vi "TempSoak_Read.vi"(0 "VISA":refnum<visa-resource-name>="TCPIP0::169.254.70.190::502::SOCKET", 1 "connection ID":refnum<k5>, 5 "error in (no error)":errorcluster, 7 "Wait(min)":dbl, 9 "stop":bool, 13 "CloseTcp(t)":bool=TRUE) -> (12 "Waveform Chart":cluster{"Value":sgl, "Value":sgl}(graph)={"Value"=27.280333, "Value"=26.223886} caption="Done!!!", 14 "visa out":refnum<visa-resource-name>, 15 "connection ID out":refnum<k5>, 19 "error out":errorcluster)   [LabVIEW 2018]
panel:
  out "x/y":dbl
  out "x-y":dbl=15.43812059999982
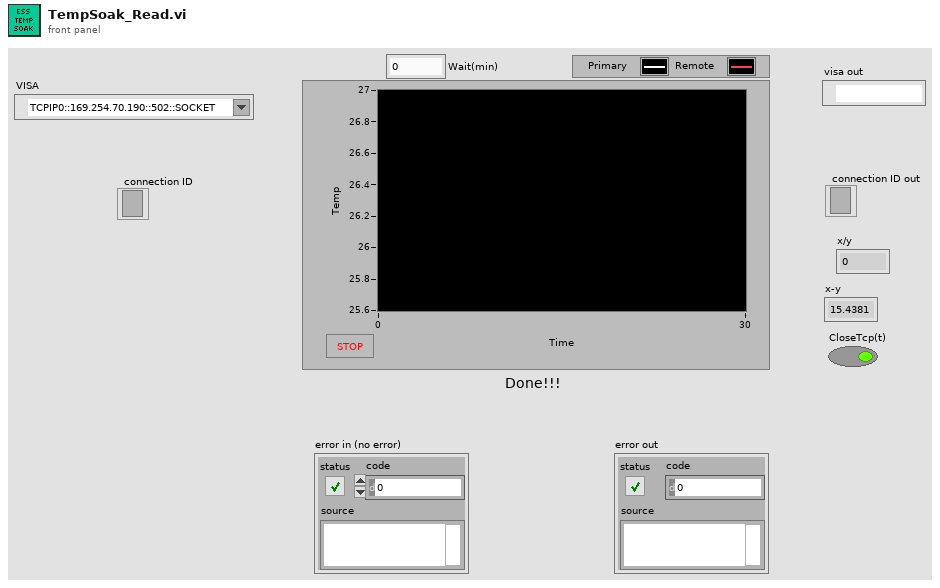
[diagram p1: front panel]
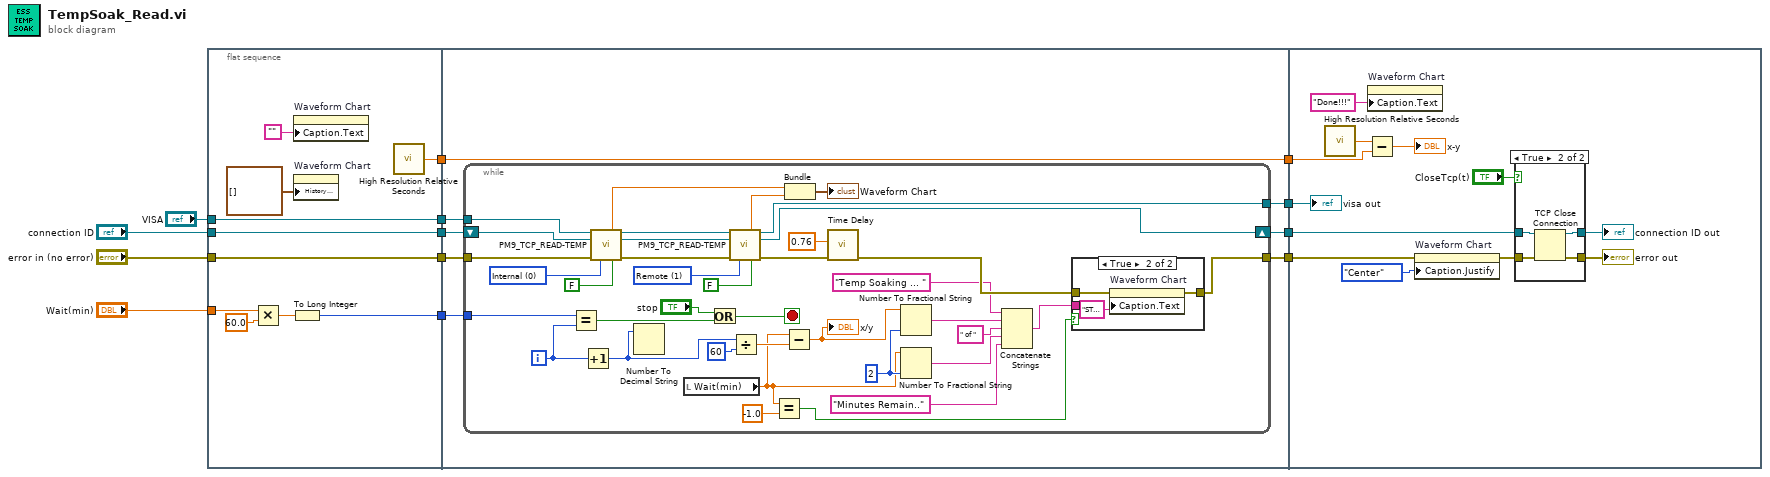
[diagram p0: block diagram]
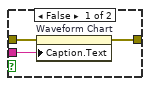
[diagram p2: hidden frame]
diagram:
  n1 = flat-sequence {
    tunnel: "connection ID" -> [w22]
    tunnel: "VISA" -> [w23]
    tunnel: [w23] -> w11
    tunnel: [w22] -> w10
    tunnel: [w21] -> w9
    tunnel: [w20] -> w7
    tunnel: "error in (no error)" -> [w20]
    tunnel: "Wait(min)" -> [w19]
    tunnel: [w16] -> w2
    tunnel: w11 -> [w31]
    tunnel: w10 -> [w30]
    tunnel: w9 -> [w29]
    tunnel: [w29] -> w8
    tunnel: w7 -> [w28]
    tunnel: [w27] -> w6
    tunnel: [w26] -> w4
    tunnel: w2 -> [w25]
    tunnel: [w24] -> w1
    tunnel: w8 -> [w86]
    tunnel: w6 -> [w80]
    tunnel: w4 -> [w84]
    tunnel: w1 -> [w76]
    frame #0 {
      n2 = Multiply(x=w19, y=60.0) -> (x*y=w17:dbl)
      n3 = To Long Integer(number=w17) -> (32bit integer=w16:i32)
      n4 = property on="Waveform Chart" class="WFChart (strict)"("Caption.Text"="") -> ()  [unwired: 2 in, 2 out]
      n5 = property on="Waveform Chart" class="WFChart (strict)"("History Data"=cluster{"Value":sgl, "Value":sgl}[] []) -> ()  [unwired: 2 in, 2 out]
      n6 = call <vilib>:"High Resolution Relative Seconds.vi"() -> ("relative seconds"=w21:dbl)
    }
    frame #1 {
      n7 = while {
        tunnel: w31 -> [w69]
        tunnel: [w62] -> w24
        shift-right: [w58] -> w26
        shift-left: w30 -> [w57]
        tunnel: w28 -> [w55]
        tunnel: [w48] -> w27
        tunnel: w25 -> [w52]
        i -> [w46]
        stop <- w51 stop-if-true
        w35 = i16 2 ("precision (6)")
        w64 = u16 1 items=["Internal", "Remote"] ("Sensor")
        w65 = u16 0 items=["Internal", "Remote"] ("Sensor")
        n8 = Equal?(x=w52, y=w46) -> (x = y?=w50:bool)
        n9 = Increment(x=w46) -> (x+1=w44:i32)
        n10 = call "PM9_TCP_READ-TEMP.vi"("VISA"=w69, "connection ID"=w57, "error in (no error)"=w55, "Sensor"=w65, "Close tcp(t)"=FALSE) -> ("Value"=w61:sgl, "visa out"=w63:refnum<visa-resource-name>, "connection ID out"=w68:refnum<k5>, "error out"=w54:errorcluster)  [unwired: 7 in]
        n11 = Number To Decimal String(number=w44) -> ()  [unwired: 1 in, 1 out]
        n12 = local read "Wait(min)"() -> (w33:dbl)
        n13 = Or(x="stop", y=w50) -> (x .or. y?=w51:bool)
        n14 = call "PM9_TCP_READ-TEMP.vi"("VISA"=w63, "connection ID"=w68, "error in (no error)"=w54, "Sensor"=w64, "Close tcp(t)"=FALSE) -> ("Value"=w60:sgl, "visa out"=w62:refnum<visa-resource-name>, "connection ID out"=w58:refnum<k5>, "error out"=w53:errorcluster)  [unwired: 7 in]
        n15 = Divide(x=w44, y=60) -> (x/y=w42:dbl)
        n16 = Equal?(x=w33, y=-1.0) -> (x = y?=w34:bool)
        n17 = Subtract(x=w33, y=w42) -> (x-y=w41:dbl)
        "x/y" <- w41
        n18 = Bundle("Value"=w61, "Value"=w60) -> (→"Waveform Chart":cluster{"Value":sgl, "Value":sgl})  [unwired: 1 in]
        n19 = call "Time Delay"("error in (no error)"=w53, "Delay Time (s)"=0.76 ("milliseconds to wait")) -> ("error out"=w49:errorcluster)  [unwired: 9 in]
        n20 = Number To Fractional String(number=w41, precision (6)=w35) -> (F-format string=w40:string)  [unwired: 2 in]
        n21 = Number To Fractional String(number=w33, precision (6)=w35) -> (F-format string=w38:string)  [unwired: 2 in]
        n22 = Concatenate Strings("Temp Soaking ... ", w40, " of " ("string"), w38, "Minutes Remain.." ("string")) -> (w36:string)
        n23 = case shown="True" w34 {
          tunnel: w49 -> [w72 w75]
          tunnel: [w71 w74] -> w48
          tunnel: w36 -> [w70 _]
          frame False {
            n24 = property on="Waveform Chart" class="WFChart (strict)"(error in=w72, "Caption.Text"=w70) -> (error out=w71:errorcluster)  [unwired: 1 in, 1 out]
          }
          frame True {
            n25 = property on="Waveform Chart" class="WFChart (strict)"(error in=w75, "Caption.Text"="STOP to Cancel" ("string")) -> (error out=w74:errorcluster)  [unwired: 1 in, 1 out]
          }
        }
      }
    }
    frame #2 {
      n26 = call <vilib>:"High Resolution Relative Seconds.vi"() -> ("relative seconds"=w87:dbl)
      n27 = Subtract(x=w87, y=w86) -> (x-y=→"x-y":dbl)
      n28 = property on="Waveform Chart" class="WFChart (strict)"("Caption.Text"="Done!!!") -> ()  [unwired: 2 in, 2 out]
      n29 = property on="Waveform Chart" class="WFChart (strict)"(error in=w80, "Caption.Justify"=enum16{"Left", "Center", "Right"}."Center" ("Caption.Justification")) -> (error out=w79:errorcluster)  [unwired: 1 in, 1 out]
      n30 = case shown="True" "CloseTcp(t)" {
        tunnel: w84 -> [w89 w93]
        tunnel: [w89 w92] -> w83
        tunnel: [w88 w91] -> w82
        tunnel: w79 -> [w88 w90]
        frame False {
        }
        frame True {
          n31 = TCP Close Connection(connection ID=w93, error in (no error)=w90) -> (connection ID out=w92:refnum<k5>, error out=w91:errorcluster)  [unwired: 1 in]
        }
      }
      "error out" <- w82
      "connection ID out" <- w83
      "visa out" <- w76
    }
  }
